vi "LEDDriver_Example.vi"() -> ()   [LabVIEW 2013]
doc: "该模板用于创建循环应用程序，通过单击“停止”按钮来结束程序的执行。单循环应用程序的VI使用轮询方式，而该模板的VI使用事件结构。"
panel:
  in  "Set Current":bool
  in  "SetStrobe Button":bool
  in  "Strobe Profile":u32[][](array[numeric])
  in  "Mode Button":bool
  in  "Normal Imax":u32[](array[numeric])
  in  "Current ModeÙ":enum32{"DISABLE", "NORMAL", "STROBE", "TRIGGER"}(ring)
  in  "Normal Current":u32(knob) max=100 scale=0.0..100.0
  in  "Current Channel":u32 max=3
  out "Serial Number:":string
  out "Handle":u32
  in  "stop":bool caption="停止"
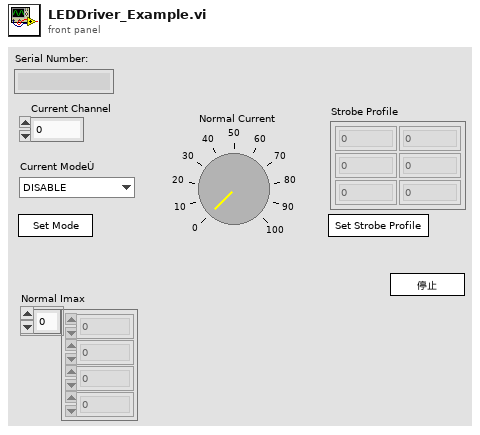
[diagram p1: front panel]
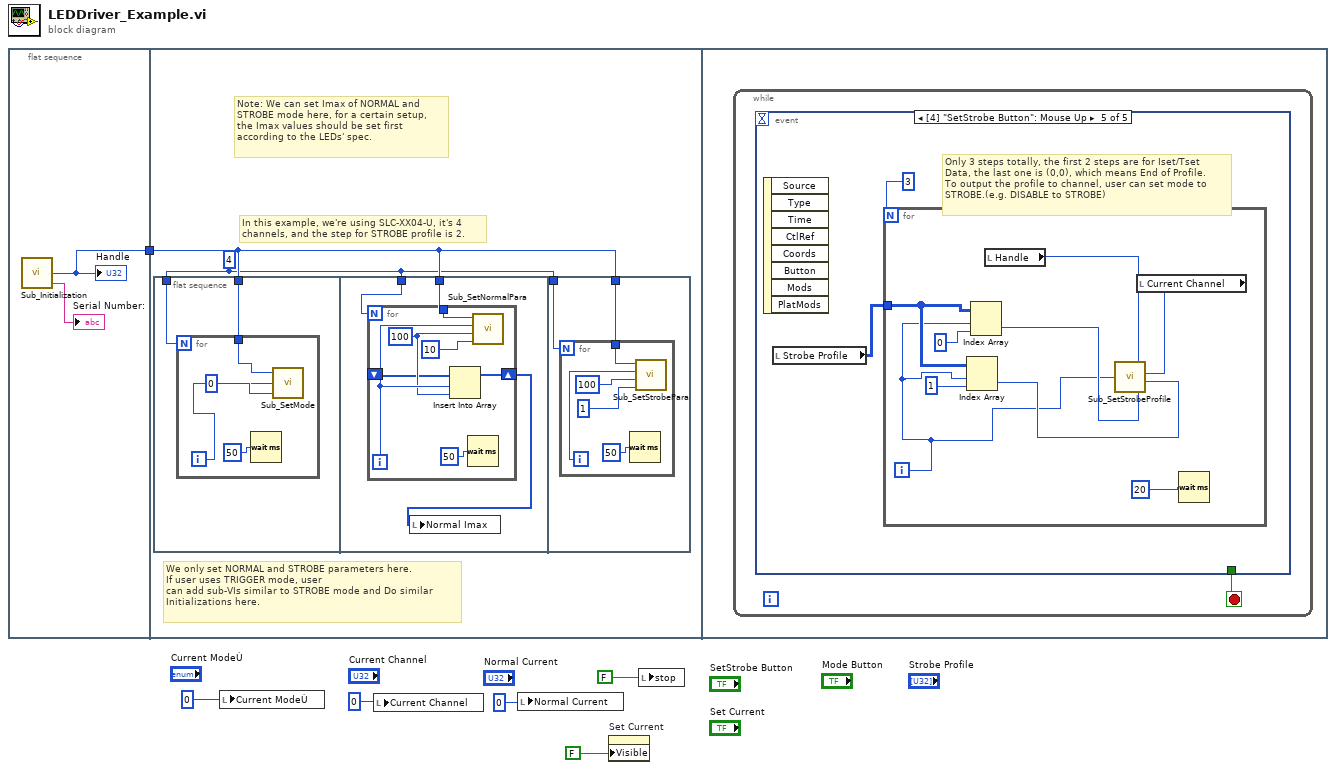
[diagram p0: block diagram]
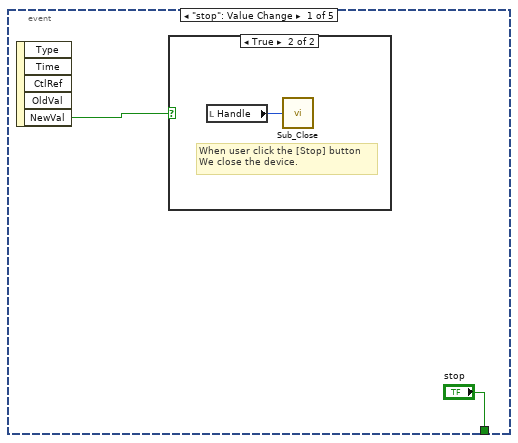
[diagram p2: hidden frame]
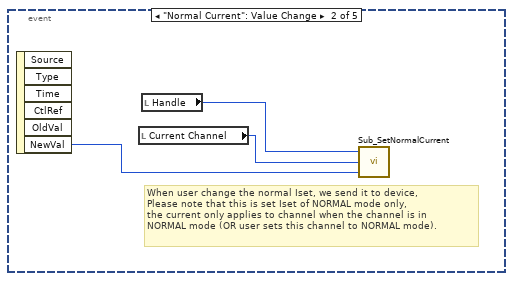
[diagram p4: hidden frame]
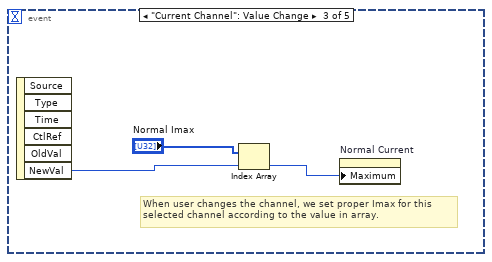
[diagram p5: hidden frame]
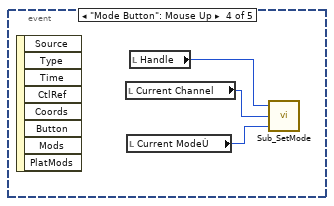
[diagram p6: hidden frame]
diagram:
  n1 = flat-sequence {
    tunnel: [w7] -> w6
    tunnel: w6 -> [w10]
    frame #0 {
      n2 = call "Sub_Initialization.vi"() -> ("SerialNumber"=→"Serial Number:":string, "DeviceHandle"=w7:u32)  [unwired: 1 out]
      "Handle" <- w7
    }
    frame #1 {
      w9 = 4
      # "In this example, we're using SLC-XX04-U, it's 4 channels, and the step for STROBE profile is 2."
      # "We only set NORMAL and STROBE parameters here.\nIf user uses TRIGGER mode, user \ncan add sub-VIs similar to STROBE mode and Do similar\nInitializations here."
      # "Note: We can set Imax of NORMAL and \nSTROBE mode here, for a certain setup,\nthe Imax values should be set first \naccording to the LEDs' spec."
      n3 = flat-sequence {
        tunnel: w10 -> [w12]
        tunnel: w9 -> [w11]
        tunnel: w10 -> [w18]
        tunnel: w9 -> [w19]
        tunnel: w9 -> [w28]
        tunnel: w10 -> [w27]
        frame #0 {
          n4 = for {
            N: w11 -> [_]
            tunnel: w12 -> [w14]
            i -> [w13]
            n5 = Wait (ms)(milliseconds to wait=50) -> ()  [unwired: 1 out]
            n6 = call "Sub_SetMode.vi"("Mode"=0, "Channel"=w13, "Device Handle"=w14) -> ()
          }
        }
        frame #1 {
          n7 = for {
            N: w19 -> [_]
            tunnel: w18 -> [w26]
            shift-right: [w21] -> w17
            shift-left: _ -> [w20]
            i -> [w23]
            w22 = 100
            n8 = Insert Into Array(array=w20, index=w23, new element=w22) -> (w21:i32[])
            n9 = Wait (ms)(milliseconds to wait=50) -> ()  [unwired: 1 out]
            n10 = call "Sub_SetNormalPara.vi"("Iset"=10, "Imax"=w22, "Channel"=w23, "Device Handle"=w26) -> ()
          }
          n11 = local write "Normal Imax"(w17) -> ()
        }
        frame #2 {
          n12 = for {
            N: w28 -> [_]
            tunnel: w27 -> [w32]
            i -> [w31]
            n13 = Wait (ms)(milliseconds to wait=50) -> ()  [unwired: 1 out]
            n14 = call "Sub_SetStrobePara.vi"("Repeat"=1, "Imax"=100, "Channel"=w31, "Device Handle"=w32) -> ()
          }
        }
      }
    }
    frame #2 {
      n15 = while {
        stop <- w34 stop-if-true
        n16 = event shown="[4] \"SetStrobe Button\": Mouse Up" {
          selector: _ -> [_ _ _ _ _]
          dyn-events: _ -> [_ _ _ _ _]
          timeout: _ -> [_ _ _ _ _]
          tunnel: ["stop" _ _ _ _] -> w34
          event "stop": Value Change {
            n17 = event-data() -> ("NewVal"=w35:bool)  [unwired: 1 in, 4 out]
            n18 = case shown="True" w35 {
              frame False {
              }
              frame True {
                # "When user click the [Stop] button\nWe close the device."
                n19 = local read "Handle"() -> (w37:u32)
                n20 = call "Sub_Close.vi"("DeviceHandle"=w37) -> ()
              }
            }
          }
          event "Normal Current": Value Change {
            # "When user change the normal Iset, we send it to device,\nPlease note that this is set Iset of NORMAL mode only,\nthe current only applies to channel when the channel is in\nNORMAL mode (OR user sets this channel to NORMAL mode)."
            n21 = event-data() -> ("NewVal"=w38:u32)  [unwired: 1 in, 5 out]
            n22 = local read "Current Channel"() -> (w39:u32)
            n23 = local read "Handle"() -> (w40:u32)
            n24 = call "Sub_SetNormalCurrent.vi"("Iset"=w38, "Channel"=w39, "Device Handle"=w40) -> ()
          }
          event "Current Channel": Value Change {
            # "When user changes the channel, we set proper Imax for this\nselected channel according to the value in array."
            n25 = event-data() -> ("NewVal"=w43:u32)  [unwired: 1 in, 5 out]
            n26 = Index Array(array="Normal Imax", index=w43) -> (element=w42:u32)
            n27 = property on="Normal Current" class="Knob (strict)"("Maximum"=w42) -> ()  [unwired: 2 in, 2 out]
          }
          event "Mode Button": Mouse Up {
            n28 = event-data() -> ()  [unwired: 1 in, 8 out]
            n29 = local read "Current Channel"() -> (w45:u32)
            n30 = local read "Current ModeÙ"() -> (w44:enum32{"DISABLE", "NORMAL", "STROBE", "TRIGGER"})
            n31 = local read "Handle"() -> (w46:u32)
            n32 = call "Sub_SetMode.vi"("Mode"=w44, "Channel"=w45, "Device Handle"=w46) -> ()
          }
          event "SetStrobe Button": Mouse Up {
            # "Only 3 steps totally, the first 2 steps are for Iset/Tset\nData, the last one is (0,0), which means End of Profile.\nTo output the profile to channel, user can set mode to\nSTROBE.(e.g. DISABLE to STROBE)"
            n33 = event-data() -> ()  [unwired: 1 in, 8 out]
            n34 = local read "Strobe Profile"() -> (w48:u32[][])
            n35 = for {
              N: 3 -> [_]
              tunnel: w48 -> [w53]
              i -> [w49]
              n36 = Index Array(array=w53, index (row)=w49, index (col)=1) -> (element=w51:u32)
              n37 = Index Array(array=w53, index (row)=w49, index (col)=0) -> (element=w54:u32)
              n38 = local read "Handle"() -> (w57:u32)
              n39 = local read "Current Channel"() -> (w56:u32)
              n40 = call "Sub_SetStrobeProfile.vi"("Step"=w49, "Device Handle"=w57, "Channel"=w56, "Tset"=w51, "Iset"=w54) -> ()
              n41 = Wait (ms)(milliseconds to wait=20) -> ()  [unwired: 1 out]
            }
          }
        }
      }
    }
  }
  n42 = local write "Current ModeÙ"(0) -> ()
  n43 = local write "Current Channel"(0) -> ()
  n44 = local write "Normal Current"(0) -> ()
  n45 = property on="Set Current" class="Bool (strict)"("Visible"=FALSE) -> ()  [unwired: 2 in, 2 out]
  n46 = local write "stop"(FALSE) -> ()
